vi "read_db_for_batch_processor.vi"(6 "Small?":bool, 7 "Update Error files?":bool, 8 "error in (no error)":errorcluster) -> (0 "error out":errorcluster, 3 "BP Array":T1[](array[typedef]) {"File Location" items=["Unknown"=-1, "Processing"=0, "Storage"=1]})   [LabVIEW 2013]
uses:
  Batch Processor/bp_cluster.ctl
  Controls/File_location.ctl
  <vilib>/addons/database/Auxilliary.llb/DB Tools Cursor Type.ctl
  <vilib>/addons/database/Connection.llb/Conn Execute.vi
  <vilib>/addons/database/Recordset.llb/Rec Fetch Recordset Data (R).vi
  <vilib>/addons/database/Recordset.llb/Rec Destroy - Connection.vi
  <vilib>/addons/database/_DB Variant To Data/Database Variant To Data.xnode
  <vilib>/addons/database/NI_Database_API.lvlib
panel:
  out "size(s)":i32
  out "SQL Query Syntax":string
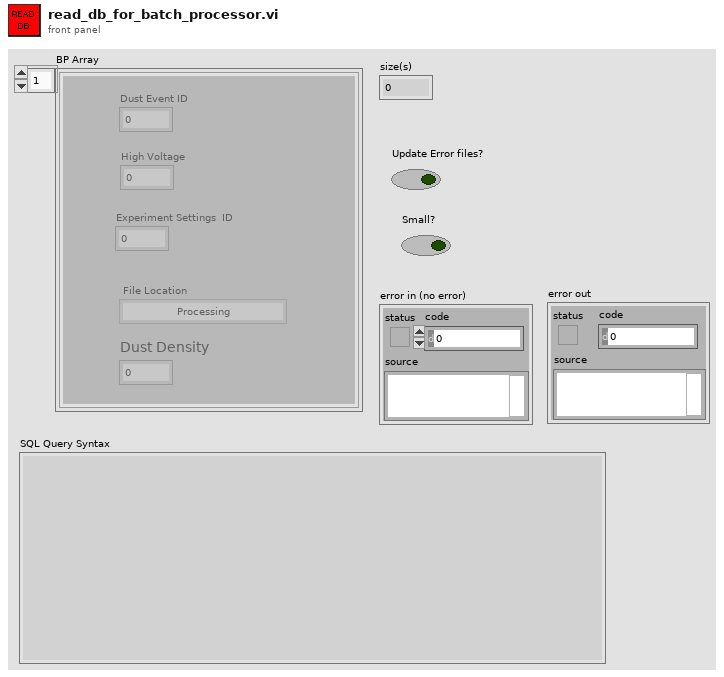
[diagram p1: front panel]
types:
  T1 = typedef "bp_cluster.ctl" = cluster{"Dust Event ID":i64, "High Voltage":sgl, "Experiment Settings  ID":i64, "File Location":T2, "Dust Density":dbl}
  T2 = typedef "File_location.ctl" = i8
  T3 = typedef "NI_Database_API.lvlib/DB Tools Cursor Type.ctl" = enum16{"forward-only", "keyset", "dynamic", "static"}
  T4 = typedef "NI_Database_API.lvlib/Conn ObjectReference.ctl" = refnum<k1>
  T5 = typedef "NI_Database_API.lvlib/Rec ObjectReference.ctl" = refnum<k1>
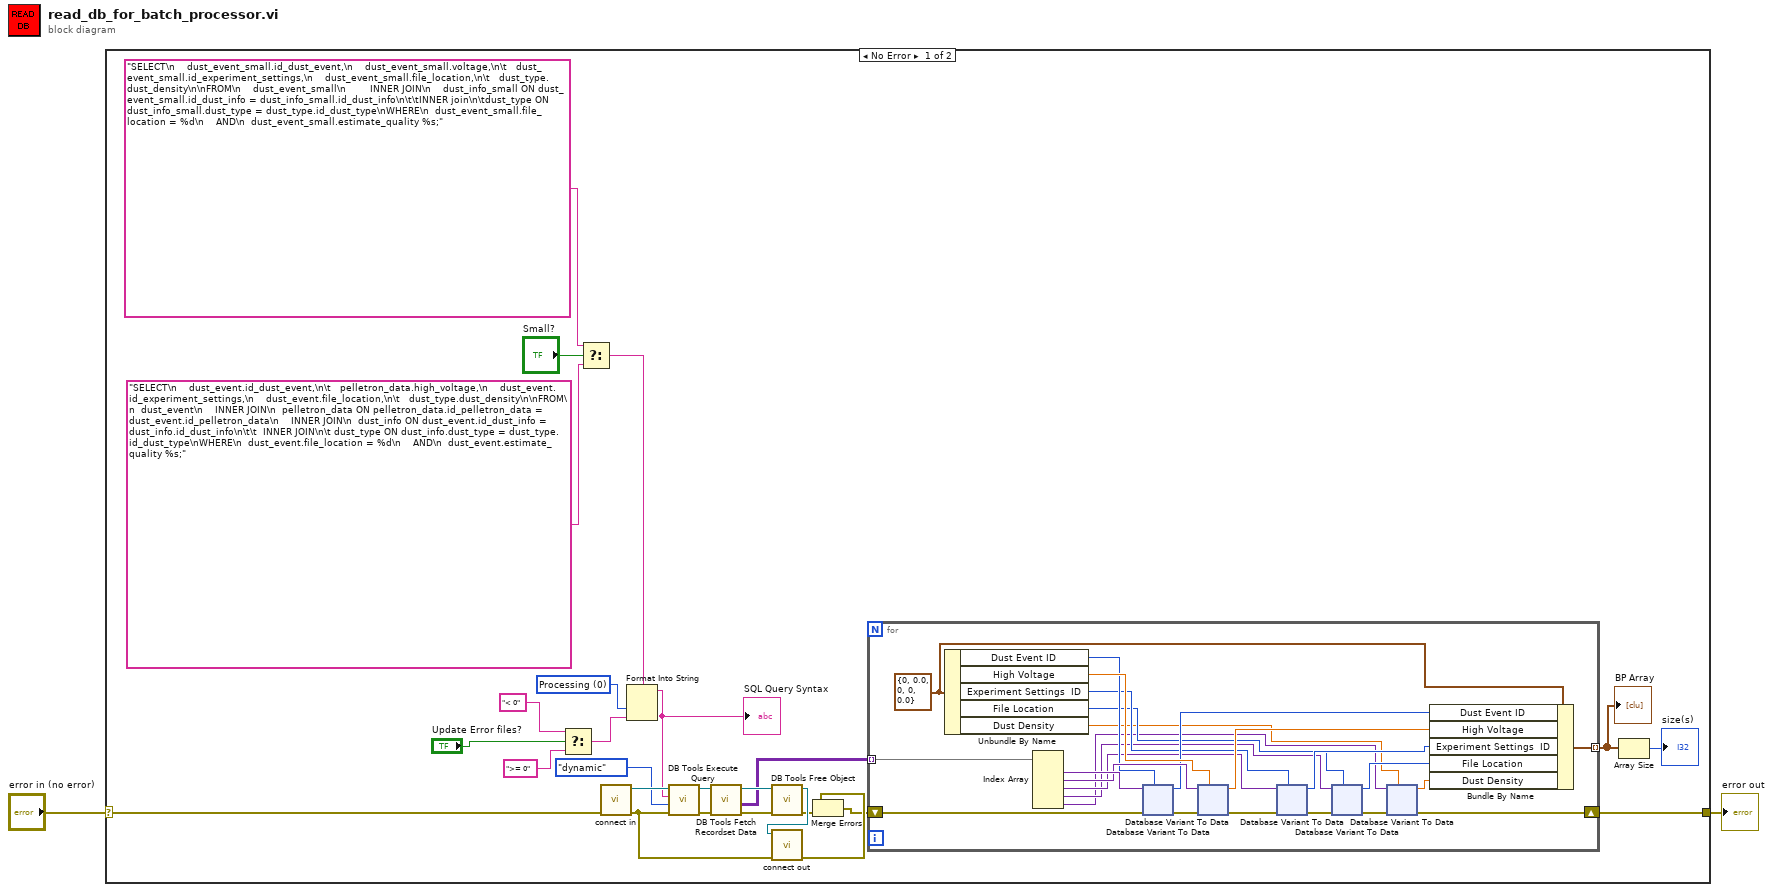
[diagram p0: block diagram]
diagram:
  n1 = case shown="No Error" "error in (no error)" {
    selector: "error in (no error)" -> [w13 w213]
    tunnel: [w7 w213] -> w1
    frame No Error {
      w5 = T2 0 items=["Unknown"=-1, "Processing"=0, "Storage"=1] ("File Location")
      n2 = Select(t="< 0", s="Update Error files?", f=">= 0") -> (s? t:f=w4:string)
      n3 = Select(t="SELECT\n    dust_event_small.id_dust_event,\n    dust_event_small.voltage,\n\t   dust_event_small.id_experiment_settings,\n    dust_event_small.file_location,\n\t   dust_type.dust_density\n\nFROM\n    dust_event_small\n        INNER JOIN\n    dust_info_small ON dust_event_small.id_dust_info = dust_info_small.id_dust_info\n\t\tINNER join\n\tdust_type ON dust_info_small.dust_type = dust_type.id_dust_type\nWHERE\n  dust_event_small.file_location = %d\n    AND\n  dust_event_small.estimate_quality %s;" ("string"), s="Small?", f="SELECT\n    dust_event.id_dust_event,\n\t   pelletron_data.high_voltage,\n    dust_event.id_experiment_settings,\n    dust_event.file_location,\n\t   dust_type.dust_density\n\nFROM\n  dust_event\n    INNER JOIN\n  pelletron_data ON pelletron_data.id_pelletron_data = dust_event.id_pelletron_data\n    INNER JOIN\n  dust_info ON dust_event.id_dust_info = dust_info.id_dust_info\n\t\t  INNER JOIN\n\t dust_type ON dust_info.dust_type = dust_type.id_dust_type\nWHERE\n  dust_event.file_location = %d\n    AND\n  dust_event.estimate_quality %s;" ("string")) -> (s? t:f=w6:string)
      n4 = call "connect in.vi"("error in (no error)"=w13) -> ("error out"=w14:errorcluster, "Database Connection"=w25:T4)  [unwired: 6 in, 1 out]
      n5 = Format Into String(format string=w6, w5, w4) -> (resulting string=w3:string)  [unwired: 2 in, 1 out]
      "SQL Query Syntax" <- w3
      n6 = call-poly <vilib>:"DB Tools Execute Query.vi"("error in (no error)"=w14, "cursor type"=DB_Tools_Cursor_Type."dynamic", "SQL query"=w3, "connection reference"=w25) -> ("error out"=w27:errorcluster, "recordset reference"=w28:T5)  [unwired: 4 in]
      n7 = call-poly <vilib>:"DB Tools Fetch Recordset Data.vi"("error in (no error)"=w27, "recordset reference"=w28) -> ("error out"=w9:errorcluster, "recordset data"=w23:variant[][], "recordset reference out"=w26:T5)  [unwired: 3 in]
      n8 = call-poly <vilib>:"DB Tools Free Object.vi"("error in (no error)"=w9, "recordset reference"=w26) -> ("error out"=w18:errorcluster, "connection reference"=w24:T4)  [unwired: 8 in]
      n9 = call "connect out.vi"("error in (no error)"=w14, "connection reference"=w24) -> ("error out"=w19:errorcluster)  [unwired: 9 in]
      n10 = Merge Errors(w19, w18) -> (w8:errorcluster)
      n11 = for {
        tunnel: w23 -> [w52] mode=indexing
        shift-right: [w49] -> w7
        shift-left: w8 -> [w51]
        tunnel: [w50] -> w21 mode=indexing
        w41 = T1 {"Dust Event ID"=0, "High Voltage"=0.0, "Experiment Settings  ID"=0, "File Location"=0, "Dust Density"=0.0} ("Batch Processing Cluster")
        n12 = Unbundle By Name(w41) -> ("Dust Event ID"=w43:i64, "High Voltage"=w44:sgl, "Experiment Settings  ID"=w39:i64, "File Location"=w34:T2, "Dust Density"=w31:dbl)
        n13 = Index Array(array=w52) -> (element #1=w48:variant, element #2=w47:variant, element #3=w40:variant, element #4=w36:variant, element #5=w30:variant)  [unwired: 5 in]
        n14 = xnode "Database Variant To Data"("database variant"=w48, "error in"=w51, "type"=w43) -> ("data"=w42:i64, "error out"=w46:errorcluster)
        n15 = xnode "Database Variant To Data"("database variant"=w47, "error in"=w46, "type"=w44) -> ("data"=w45:sgl, "error out"=w37:errorcluster)
        n16 = xnode "Database Variant To Data"("database variant"=w40, "error in"=w37, "type"=w39) -> ("data"=w38:i64, "error out"=w35:errorcluster)
        n17 = xnode "Database Variant To Data"("database variant"=w36, "error in (no error)"=w35, "type"=w34) -> ("data"=w33:T2, "error out"=w32:errorcluster)
        n18 = xnode "Database Variant To Data"("database variant"=w30, "error in"=w32, "type"=w31) -> ("data"=w29:dbl, "error out"=w49:errorcluster)
        n19 = Bundle By Name(cluster=w41, "Dust Event ID"=w42, "High Voltage"=w45, "Experiment Settings  ID"=w38, "File Location"=w33, "Dust Density"=w29) -> (w50:T1)
      }
      "BP Array" <- w21
      n20 = Array Size(array=w21) -> (size(s)=→"size(s)":i32)
    }
    frame Error {
    }
  }
  "error out" <- w1
